vi "Set Goal D.vi"(11 "GIC Input":T1={"     Use ?\nOff       On"=[FALSE, TRUE, FALSE, TRUE], "Mode:"=FALSE, "Extra Port"="", "Hokuyo Port"="COM7", "Tx Prop  Port"="COM6", "Compass Port"="", "GPS Port"="", "Num of WPs"=0, "WP Lats and Longs"={"WP Lats"=[], "WP Longs"=[]}, "Obst Lats and Longs"={"Obst Lats"=[], "Obst Longs"=[]}, "Parameters"=[], "GPS Data"=[], "Compass"=0.0, "LMS Vector"=[], "Vision Vector"=[], "Direction Cmd"=0.0, "Speed Cmd"=0.0, "WP Vector"=[], "WP Number"=0, "Extra"=0, "SW Map"=[], "Path Cluster"={"Path x node"=[], "Path y node"=[]}, "Sim Course"=[]} {"Obst Lats and Longs"."Obst Longs" format="%#_8g"; "Obst Lats and Longs"."Obst Lats" format="%#_8g"}) -> (3 "GIC Output":T1={"     Use ?\nOff       On"=[FALSE, TRUE, FALSE, TRUE], "Mode:"=FALSE, "Extra Port"="", "Hokuyo Port"="COM7", "Tx Prop  Port"="COM6", "Compass Port"="", "GPS Port"="", "Num of WPs"=0, "WP Lats and Longs"={"WP Lats"=[], "WP Longs"=[]}, "Obst Lats and Longs"={"Obst Lats"=[], "Obst Longs"=[]}, "Parameters"=[], "GPS Data"=[], "Compass"=0.0, "LMS Vector"=[], "Vision Vector"=[], "Direction Cmd"=0.0, "Speed Cmd"=0.0, "WP Vector"=[], "WP Number"=0, "Extra"=0, "SW Map"=[], "Path Cluster"={"Path x node"=[], "Path y node"=[]}, "Sim Course"=[]} {"Obst Lats and Longs"."Obst Longs" format="%#_8g"; "Obst Lats and Longs"."Obst Lats" format="%#_8g"})   [LabVIEW 2014]
panel:
  out "tes10":dbl
  out "tes9":dbl
  out "tes8":dbl
  out "tes7":dbl
  out "tes6":dbl
  out "tes5":dbl
  out "tes4":dbl
  out "tes3":dbl
  out "tes2":dbl
  out "tes1":dbl
  out "Slant Conf":dbl
  out "Slant":dbl
  out "test 2":dbl
  out "tp":dbl
  out "wp vector":dbl[](array[numeric])
  out "test 1":dbl
  out "goal y":dbl
  out "goal x":dbl
  out "Test Output SWMap":dbl[][](array[numeric])
  # "Set Goal D"
  # "Input:"
  # "Output:"
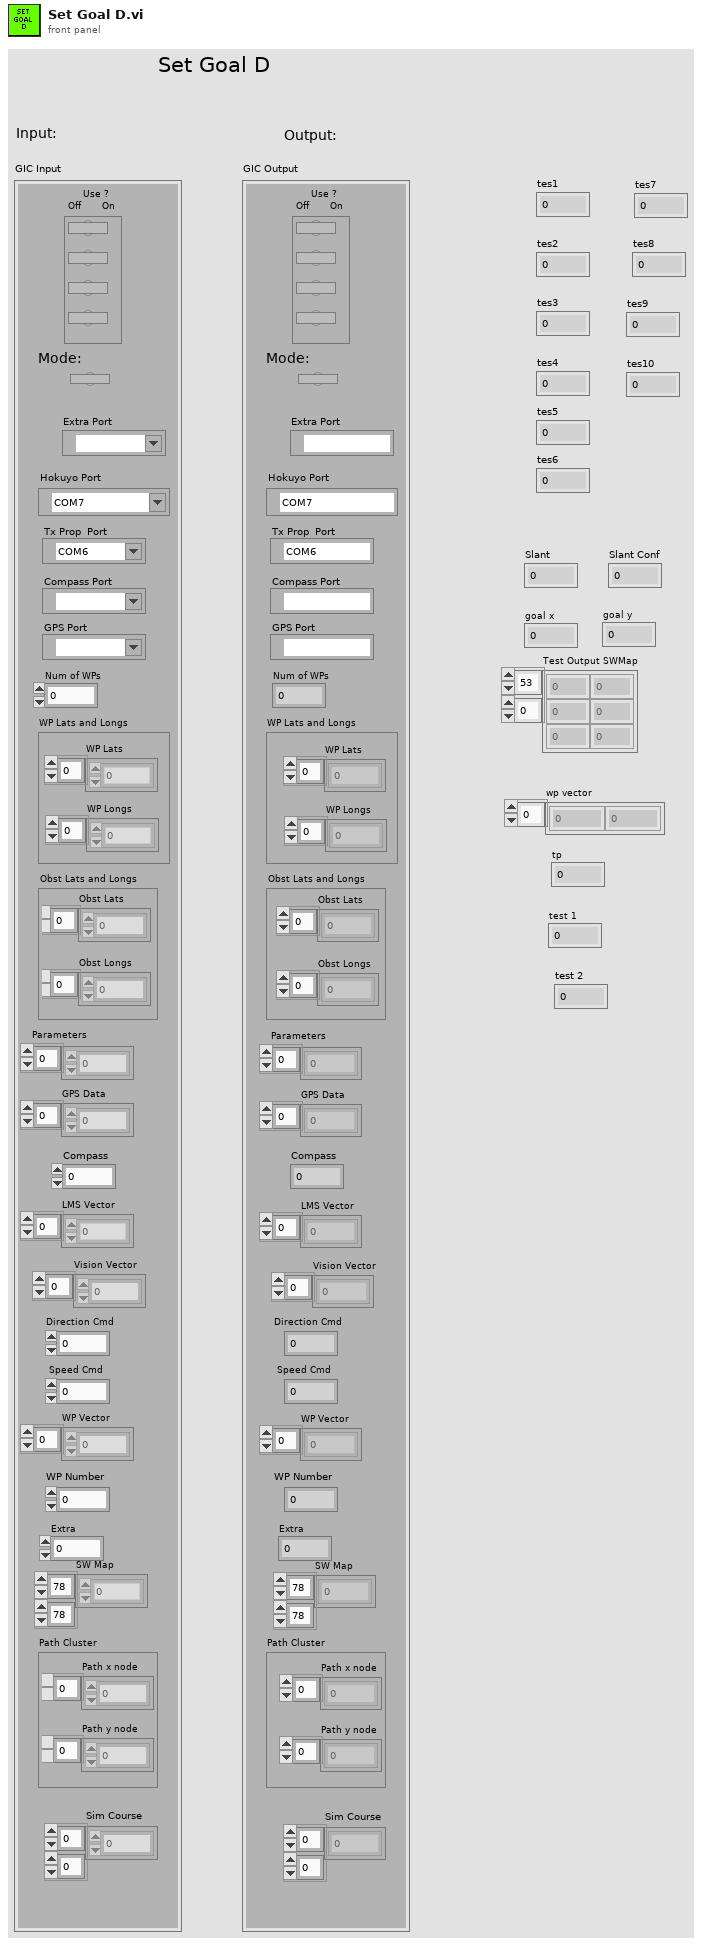
[diagram p1: front panel]
types:
  T1 = cluster{"     Use ?\nOff       On":bool[], "Mode:":bool, "Extra Port":refnum<visa-resource-name>, "Hokuyo Port":refnum<visa-resource-name>, "Tx Prop  Port":refnum<visa-resource-name>, "Compass Port":refnum<visa-resource-name>, "GPS Port":refnum<visa-resource-name>, "Num of WPs":i16, "WP Lats and Longs":cluster{"WP Lats":dbl[], "WP Longs":dbl[]}, "Obst Lats and Longs":cluster{"Obst Lats":dbl[], "Obst Longs":dbl[]}, "Parameters":dbl[], "GPS Data":dbl[], "Compass":dbl, "LMS Vector":dbl[], "Vision Vector":dbl[], "Direction Cmd":dbl, "Speed Cmd":dbl, "WP Vector":dbl[], "WP Number":i32, "Extra":i16, "SW Map":i32[][], "Path Cluster":cluster{"Path x node":dbl[], "Path y node":dbl[]}, "Sim Course":i8[][]}
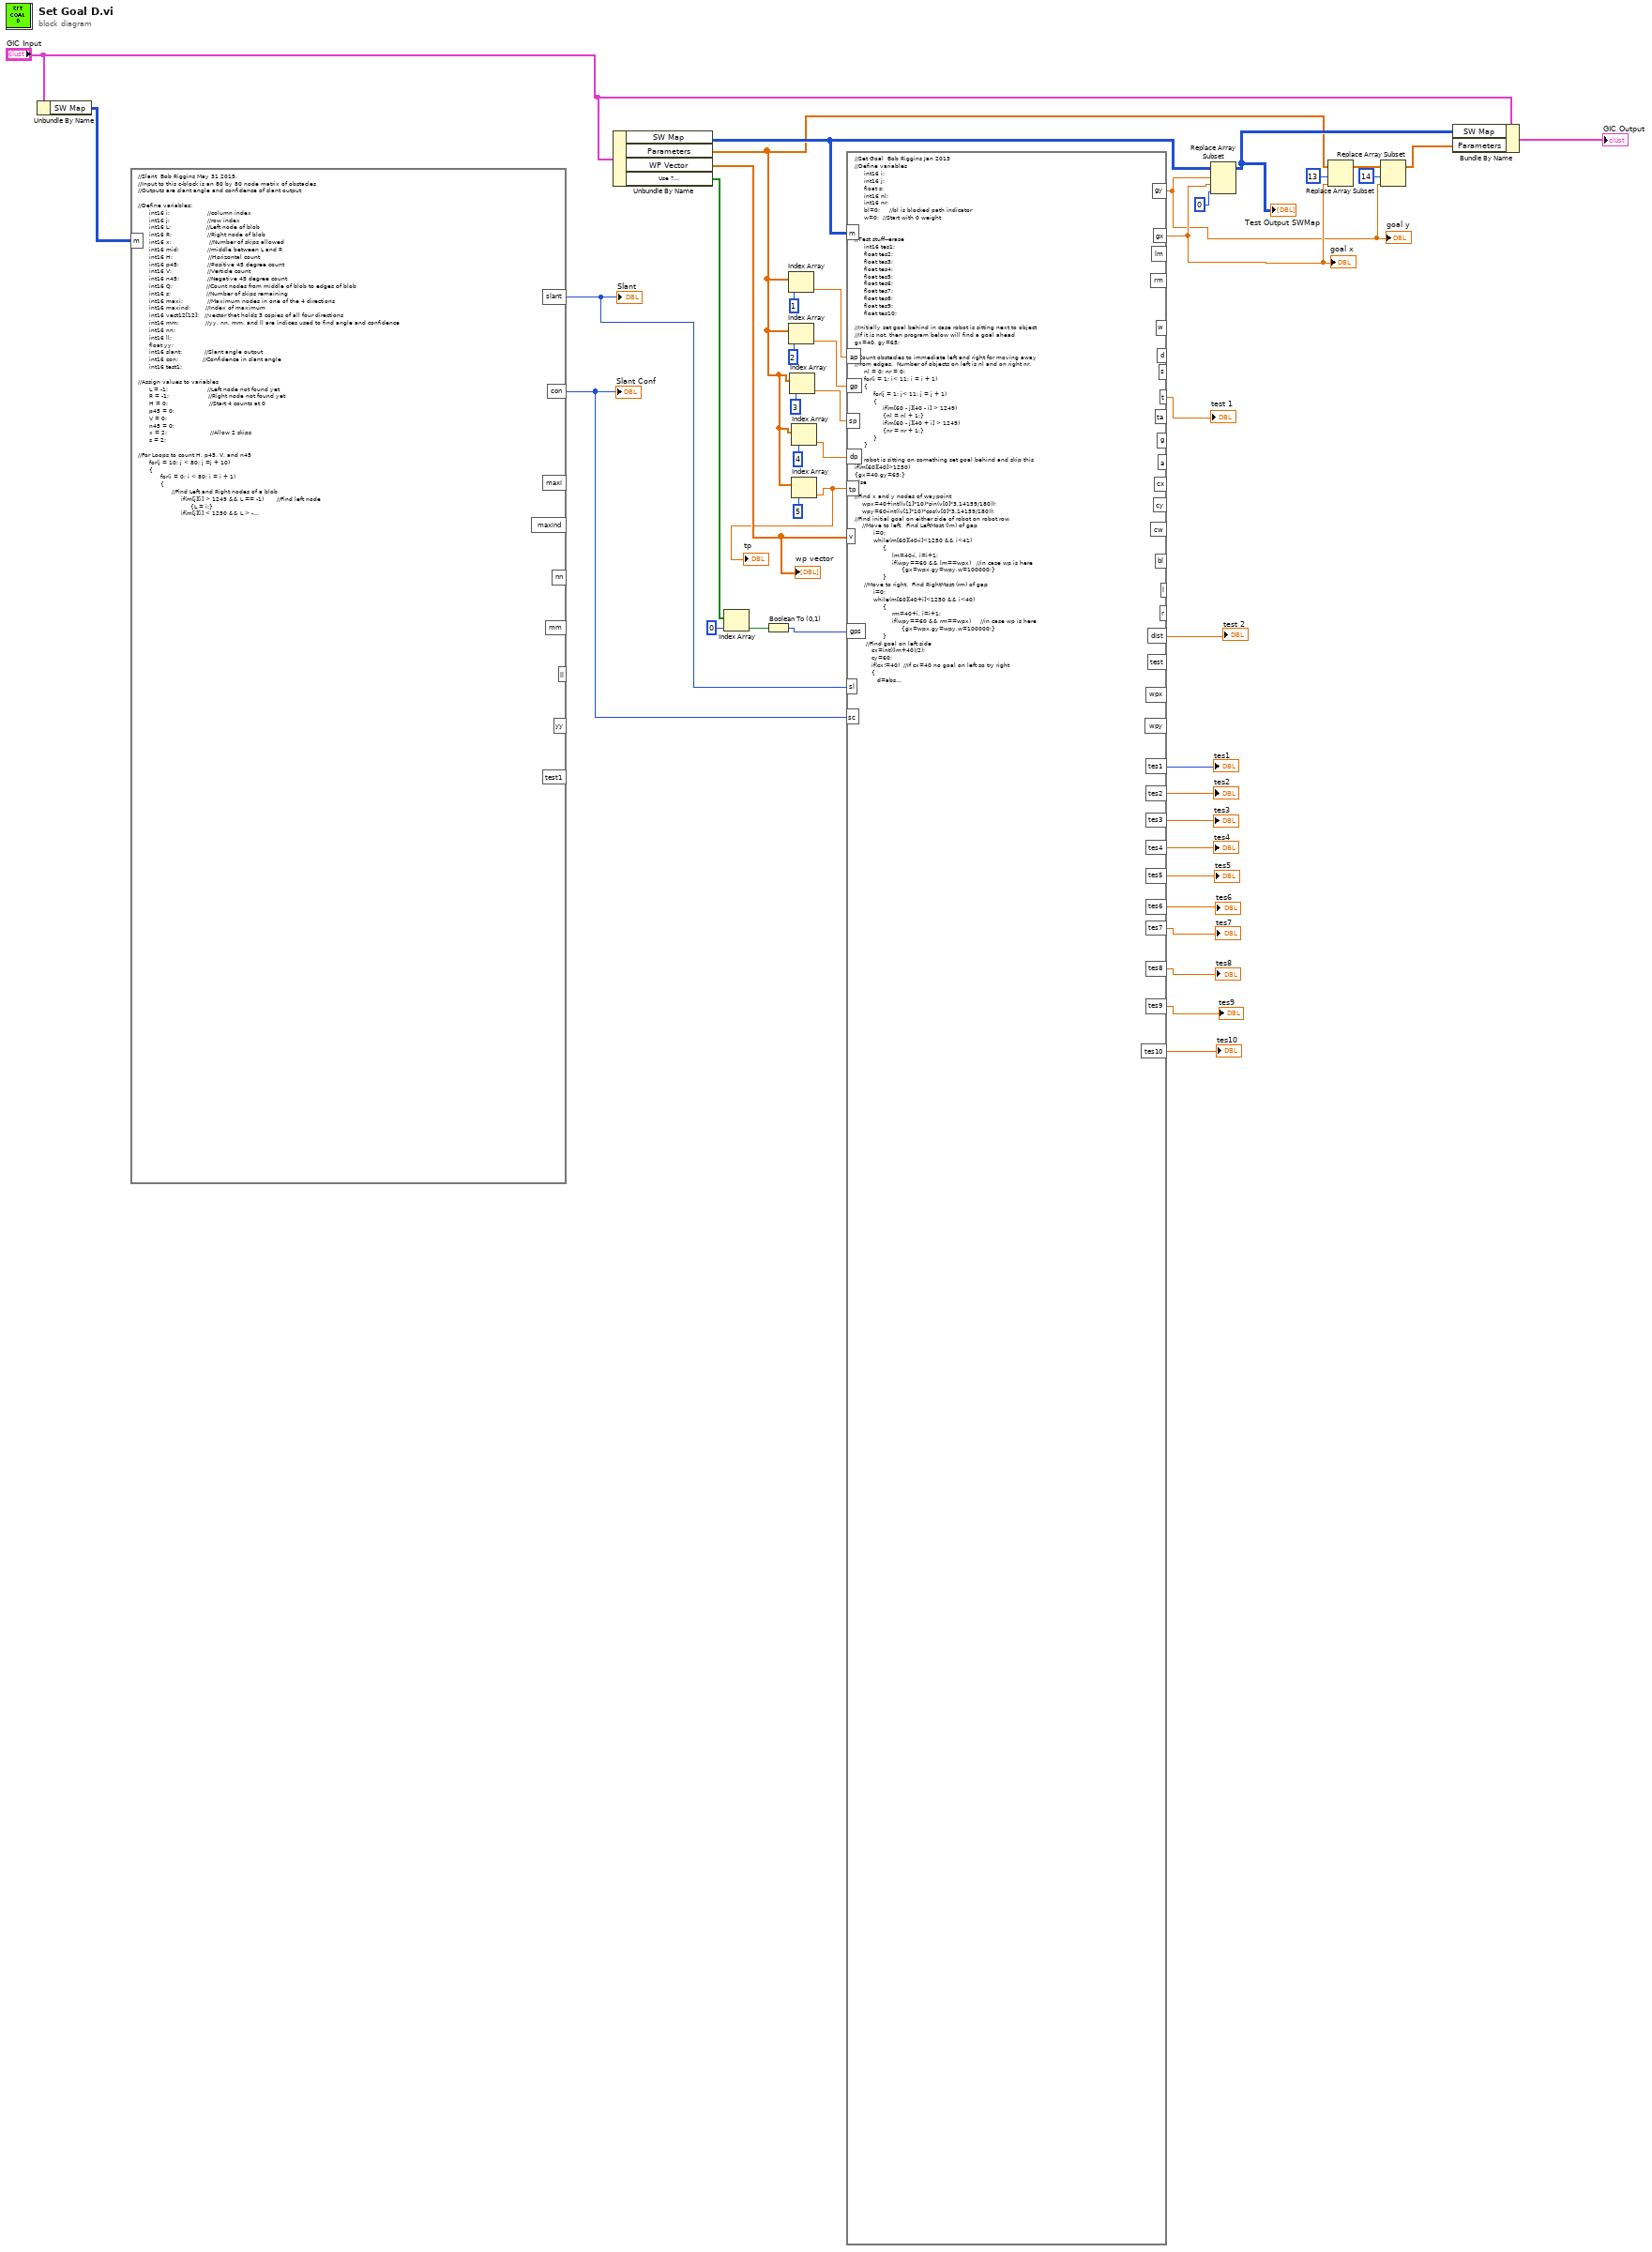
[diagram p0: block diagram]
diagram:
  n1 = Unbundle By Name("GIC Input") -> ("SW Map"=w13:i32[][])
  n2 = formula code="//Slant  Bob Riggins May 31 2015.  \n//Input to this c-block is an 80 by 80 node matrix of obstacles\n//Outputs are slant angle and confidence of slant output\n\n//Define variables:\n      int16 i;                    //column index\n      int16 j;                    //row index\n      int16 L;                   //Left node of blob\n      int16 R;                   //Right node of blob\n      int16 x;                    //Number of skips allowed\n      int16 mid;               //middle between L and R\n      int16 H;                   //Horizontal count\n      int16 p45;               //Positive 45 degree count\n      int16 V;                   //Verticle count\n      int16 n45;               //Negative 45 degree count\n      int16 Q;                  //Count nodes from middle of blob to edges of blob\n      int16 s;                   //Number of skips remaining\n      int16 maxi;             //Maximum nodes in one of the 4 directions\n      int16 maxind;        //Index of maximum\n      int16 vect12[12];   //vector that holds 3 copies of all four directions\n      int16 mm;              //yy, nn, mm, and ll are indices used to find angle and confidence\n      int16 nn;\n      int16 ll;\n      float yy;\n      int16 slant;            //Slant angle output\n      int16 con;             //Confidence in slant angle\n      int16 test1;\n\n//Assign values to variables\n      L = -1;                     //Left node not found yet\n      R = -1;                     //Right node not found yet\n      H = 0;                      //Start 4 counts at 0\n      p45 = 0;\n      V = 0;\n      n45 = 0;\n      x = 2;                       //Allow 2 skips\n      s = 2;\n\n//For Loops to count H, p45, V, and n45\n      for(j = 10; j < 80; j =j + 10)\n      {\n            for(i = 0; i < 80; i = i + 1)\n            {\n                  //Find Left and Right nodes of a blob\n                       if(m[j][i] > 1249 && L == -1)       //Find left node\n                            {L = i;}\n                       if(m[j][i] < 1250 && L > -1 && s == 0)          //Find right node\n                            {R = i - 1 - x;} \n                       if(m[j][i] <1250 && L > -1 && s > 0)         //Allow for skips\n                            {s = s - 1;}\n                       if(i == 79 && m[j][i] > 1249 && L == -1)      //single node at edge\n                       {                                                                            //define L and R there\n                             L == 79;\n                             R == 79;\n                       }       \n                       if(i == 79 && m[j][i] > 1249 && L > -1)       //blob at edge (L found)\n                            {R = 79;}   \n                       if(i == 79 && m[j][i] < 1250 && L > -1)       //blob at edge (L found)\n                            {R = 78;}\n\n                       if(L > -1 && R > -1)         //If L and R exist then start counting from mid\n                       {\n                            H = H + (R - L);                         //Updated H\n                            if(j==10)\n                                 {test1 = R;}\n                            mid = int((L + R)/2);                //Set up middle of blob for counting\n                            L = -1;\n                            R = -1;\n                            s = x;\n                            Q = 1; \n                \n                       //Count N45 (negative 45 degrees thru mid of blob)\n                            while (s > 0 && j + Q < 80 && mid + Q < 80)\n                                {\n                                     while (m[j + Q][mid + Q] > 1249)    //Count down and to right\n                                          {\n                                               n45 = n45 + 1;\n                                               s = x;\n                                               Q = Q + 1;\n                                          }\n                                     while (m[j + Q][mid + Q] < 1250 && s > 0)   //Allow x skips\n                                          {\n                                               n45 = n45 + 1;\n                                               s = s - 1;\n                                               Q = Q + 1;\n                                          }\n                                }     //end of while loop for counting n45 down and to right\n                                n45 = n45 - x;\n                                s = x;\n                                Q = 1;\n\n                                while (s > 0 && j - Q > -1 && mid - Q > -1)\n                                {\n                                     while (m[j - Q][mid - Q] > 1249)    //Count up and to left\n                                          {\n                                               n45 = n45 + 1;\n                                               s = x;\n                                               Q = Q + 1;\n                                          }\n                                     while (m[j - Q][mid - Q] < 1250 && s > 0)   //Allow x skips\n                                          {\n                                               n45 = n45 + 1;\n                                               s = s - 1;\n                                               Q = Q + 1;\n                                          }\n                                }     //end of while loop for counting n45 up and to left\n                                n45 = n45 - x;\n                                s = x;\n                                Q = 1;\n\n                       //Count V (verticle thru mid of blob)\n                            while (s > 0 && j + Q < 80)\n                                {\n                                     while (m[j + Q][mid] > 1249)    //Count down from mid\n                                          {\n                                               V = V + 1;\n                                               s = x;\n                                               Q = Q + 1;\n                                          }\n                                     while (m[j + Q][mid] < 1250 && s > 0)   //Allow x skips\n                                          {\n                                               V = V + 1;\n                                               s = s - 1;\n                                               Q = Q + 1;\n                                          }\n                                }     //end of while loop for counting V down\n                                V = V - x;\n                                s = x;\n                                Q = 1;\n\n                                while (s > 0 && j - Q > -1)\n                                {\n                                     while (m[j - Q][mid] > 1249)    //Count up\n                                          {\n                                               V = V + 1;\n                                               s = x;\n                                               Q = Q + 1;\n                                          }\n                                     while (m[j - Q][mid] < 1250 && s > 0)   //Allow x skips\n                                          {\n                                               V = V + 1;\n                                               s = s - 1;\n                                               Q = Q + 1;\n                                          }\n                                }     //end of while loop for counting V up\n                                V = V - x;\n                                s = x;\n                                Q = 1;\n\n                       //Count p45 (positive 45 degrees thru mid of blob)\n                            while (s > 0 && j + Q < 80 && mid - Q > -1)\n                                {\n                                     while (m[j + Q][mid - Q] > 1249)    //Count down and to left\n                                          {\n                                               p45 = p45 + 1;\n                                               s = x;\n                                               Q = Q + 1;\n                                          }\n                                     while (m[j + Q][mid - Q] < 1250 && s > 0)   //Allow x skips\n                                          {\n                                               p45 = p45 + 1;\n                                               s = s - 1;\n                                               Q = Q + 1;\n                                          }\n                                }     //end of while loop for counting p45 down and to left\n                                p45 = p45 - x;\n                                s = x;\n                                Q = 1;\n\n                                while (s > 0 && j - Q > -1 && mid + Q < 80)\n                                {\n                                     while (m[j - Q][mid + Q] > 1249)    //Count up and to right\n                                          {\n                                               p45 = p45 + 1;\n                                               s = x;\n                                               Q = Q + 1;\n                                          }\n                                     while (m[j - Q][mid + Q] < 1250 && s > 0)   //Allow x skips\n                                          {\n                                               p45 = p45 + 1;\n                                               s = s - 1;\n                                               Q = Q + 1;\n                                          }\n                                }     //end of while loop for counting p45 up and to right\n                                p45 = p45 - x;\n                                s = x;\n                                Q = 1;\n\n                       }                                                    //end of IF for counts for blob\n            }                                    //end of FOR for i\n      }                                          //end of FOR for j\n      \n      //Now have H, p45, V, n45.  Find slan and con  (slant angle and confidence)\n            maxi = H;                                   //Initialize process of finding maximum direction\n            maxind = 0;\n            if(p45 > maxi)\n            {\n                 maxi = p45;\n                 maxind = 1;\n            }\n            if(V > maxi)\n            {\n                 maxi = V;\n                 maxind = 2;\n            }\n            if(n45 > maxi)\n            {\n                 maxi = n45;\n                 maxind = 3;\n            }                                                    //now, max value of 4 directions in maxi\n                                                                 //maxind is index of direction of max\n\n            for(i = 0; i < 3; i = i + 1)            //Next, make vect12, 3 copies of 4 directions\n            {\n                 vect12[4*i] = H;\n                 vect12[4*i + 1] = p45;\n                 vect12[4*i + 2] = V;\n                 vect12[4*i + 3] = n45;\n            }\n           \n            if(maxi != 0)\n            {\n                 nn = vect12[maxind - 1];                          //Use max direction and \"pull\" off to sides\n                 mm = vect12[maxind + 1];\n                 ll = vect12[maxind + 2];\n                 yy = (mm - nn)/(maxi + mm + mm);\n                 con = (1 - (ll/maxi)) * 100;                                    //Confidence of slant calculation\n\n                 if(maxind == 0)                                         //Find slant angle\n                    {slant = 45 * yy;}\n                 if(maxind == 1)                                         \n                    {slant = 45 * (1 - yy);}\n                 if(maxind == 2)                                         \n                    {slant = (45 * (1 - yy)) - 45;}\n                 if(maxind == 3)                                         \n                    {slant = -45 * (1 + yy);}\n             }\n\n             if(maxi == 0)\n             {\n                  slant = 0;\n                  con = 0;\n             }"("m"=w13) -> ("slant"=w5:i16, "con"=w4:i16)  [unwired: 7 out]
  "Slant" <- w5
  "Slant Conf" <- w4
  n3 = Unbundle By Name("GIC Input") -> ("SW Map"=w40:i32[][], "Parameters"=w30:dbl[], "WP Vector"=w23:dbl[], "Use ?\nOff       On"=w21:bool[])
  "wp vector" <- w23
  n4 = Index Array(array=w21, index=0) -> (element=w19:bool)
  n5 = Boolean To (0,1)(Boolean=w19) -> (0, 1=w18:i16)
  n6 = Index Array(array=w30, index=1) -> (element=w39:dbl)
  n7 = Index Array(array=w30, index=2) -> (element=w36:dbl)
  n8 = Index Array(array=w30, index=3) -> (element=w34:dbl)
  n9 = Index Array(array=w30, index=4) -> (element=w32:dbl)
  n10 = Index Array(array=w30, index=5) -> (element=w22:dbl)
  "tp" <- w22
  n11 = formula code="//Set Goal  Bob Riggins Jan 2013\n//Define variables\n     int16 i;\n     int16 j;\n     float s;\n     int16 nl;\n     int16 nr;\n     bl=0;     //bl is blocked path indicator\n     w=0;  //Start with 0 weight\n     \n\n//Test stuff--erase\n     int16 tes1;\n     float tes2;\n     float tes3;\n     float tes4;\n     float tes5;\n     float tes6;\n     float tes7;\n     float tes8;\n     float tes9;\n     float tes10;\n\n//Initially set goal behind in case robot is sitting next to object\n//If it is not, then program below will find a goal ahead\ngx=40, gy=65;\n\n//Count obstacles to immediate left and right for moving away\n//from edges.  Number of objects on left is nl and on right nr.\n     nl = 0; nr = 0;\n     for(i = 1; i< 11; i = i + 1)\n     {\n          for(j = 1; j< 11; j = j + 1)\n          {\n               if(m[60 - j][40 - i] > 1249)\n               {nl = nl + 1;}\n               if(m[60 - j][40 + i] > 1249)  \n               {nr = nr + 1;}\n          }\n     }   \n\n//If robot is sitting on something set goal behind and skip this\nif(m[60][40]>1250)\n{gx=40,gy=65;}\nelse\n{\n//Find x and y nodes of waypoint\n    wpx=40+int((v[1]*10)*sin(v[0]*3.14159/180));\n    wpy=60-int((v[1]*10)*cos(v[0]*3.14159/180));\n//Find initial goal on either side of robot on robot row\n    //Move to left.  Find LeftMost (lm) of gap\n          i=0;\n          while(m[60][40-i]<1250 && i<41)\n               {\n                    lm=40-i, i=i+1;\n                    if(wpy==60 && lm==wpx)   //in case wp is here\n                         {gx=wpx,gy=wpy,w=100000;}\n               }\n     //Move to right.  Find RightMost (rm) of gap\n          i=0;\n          while(m[60][40+i]<1250 && i<40)\n               {\n                    rm=40+i, i=i+1;\n                    if(wpy==60 && rm==wpx)     //in case wp is here\n                         {gx=wpx,gy=wpy,w=100000;}\n               }\n      //Find goal on left side\n         cx=int((lm+40)/2);\n         cy=60;\n         if(cx!=40)  //If cx=40 no goal on left so try right\n         {\n            d=abs(cx-40)*v[1]/100; //d depends on wp dist\n            if(d>100)\n                                    {d = 100;}\n            s=0;  //slant is not allpicable initially\n            ta=v[0]*.01745;  //Angle to waypoint (target)\n            //WP angle dot product reduces for cy=60 to:\n            t=((((sin(ta)*(cx-40))/abs(cx-40))+1)*50)/v[1];  //0-100\n            //g=(40-lm)*1.25;   //gap size 0-100\n            g = 0;\n            //a=0;  //not applicable initially\n            //a=(100-(abs(cx-40)*2.5))*(100-tp)/100;\n\n            a = 0;\n            if(nl > nr && cx > 40 && cy > 30) \n                 {a = 100;}\n            if(nl < nr && cx < 40 && cy > 30) \n                 {a = 100;}\n                       \n            cw=(d*dp)+(s*sp)+(t*tp)+(g*gp)+(a*ap);\n            if(cw>w)       //this is new weight if better than old\n              {w=cw, gx=cx, gy=cy;\n                tes1 = cx; tes2 = v[1]; tes3 = ta; tes4 = t; tes5 = g; tes6 = a;\n                tes7 = d;}\n         }\n      //Note if cx=40  no good on left so keep w=0 and try right\n      //Find candidate goal on right side\n         cx=int((40+rm)/2);  \n         cy=60;\n         if(cx!=40)  //If cx=40 no goal on right so dont even try\n         {\n              d=abs(cx-40)*v[1]/100; \n              if(d>100)\n                                    {d = 100;} \n              s=0;  //slant is not allpicable initially\n              ta=v[0]*.01745;  //Angle to waypoint (target)\n              //WP angle dot product reduces for gy=60 to:\n              t=((((sin(ta)*(cx-40))/abs(cx-40))+1)*50)/v[1];  //0-100\n              //g=(rm-40)*1.25;   //gap size 0-100\n              g = 0;\n              //a=0;  //not applicable initially\n              //a=(100-(abs(cx-40)*2.5))*(100-tp)/100;\n              a = 0;\n              if(nl > nr && cx > 40 && cy > 30) \n                  {a = 100;}\n              if(nl < nr && cx < 40 && cy > 30) \n                  {a = 100;}\n              cw=(d*dp)+(s*sp)+(t*tp)+(g*gp)+(a*ap);\n              if(cw>w)       //change goal if the right is better\n                   {w=cw, gx=cx, gy=cy;\n                     tes1 = cx; tes2 = v[1]; tes3 = ta; tes4 = t; tes5 = g; tes6 = a;\n                     tes7 = d;} \n         }    \n\n//Main Loop, move up row by row checking candidates\n//Candidate goals are midpoints and both edges of all gaps\n     cy=60;\n     while(cy>0&&bl==0)\n     {\n      //start scout one row up and 1 to left unless on edge\n           if(lm==0)\n                {cx=0;}\n           else\n                {cx=lm-1;}\n           cy=cy-1; \n      //move scout to right until on clear node\n           while(m[int(cy)][int(cx)]>1249 && cx<80)\n                {cx=cx+1;}\n           if(cx==80||cx>rm+1)\n            {bl=1;  }   //means this row is blocked--can quit looking  \n      //move scout to left until on occupied node--make new lm\n           while(m[int(cy)][int(cx)]<1250 && cx>0 && bl==0)\n                {\n                    cx=cx-1;\n                    if(cy==wpy && cx==wpx)     //in case wp is here\n                         {gx=wpx,gy=wpy,w=100000;}\n                }\n           cx=cx+1;\n           lm=cx;       //new lm\n           l=lm;              //l is left of first gap on row\n      //Find all gaps on row by finding l and r of each\n      //l of first gap already found above (l=lm)\n           i=lm;  //start scout i at lm\n           while(i<80 && bl==0)   //move across row to find all gaps  \n                {\n                     while(m[int(cy)][i]<1250 && i<80)\n                          {\n                               i=i+1;\n                               if(cy==wpy && i==wpx)     //in case wp is here\n                                    {gx=wpx,gy=wpy,w=100000;}\n                          }\n                     if(i==80)\n                          {rm=79, r=rm;}\n                     else\n                          {r=i-1;}   //we now have l and r of this gap\n\n                     //Next search for best goal so far in this gap\n                     //Set goal only in middlepoint unless on edge and\n                     //unless use gps\n\n                     if(cy==0 && gps==1)\n                     {\n                          for(cx=l;cx<=r;cx=cx+1)\n                          {\n                               dist=((cx-40)**2+(cy-60)**2)**.5;\n                               d=dist*v[1]/100; \n                               if(d>100)\n                                    {d = 100;}\n                               ta=v[0]*.01745;  //Angle to waypoint (target)\n                               t=(((((cx-40)*sin(ta)+(60-cy)*cos(ta))/dist)+1)*50)/v[1];\n                               //g=(r-l)*1.25;   //gap size 0-100\n                               if(r-l<=60)\n                                    {g=100-(abs(r-l-30)*3.33);}\n                               else\n                                    {g=0;}\n                               a=0;  //not applicable initially \n                               //a=(100-(abs(cx-40)*2.5))*(100-tp)/100;\n                               //a = (60 - cy)*v[1]/dist;\n                               s=((((cx-40)*sin(sl*3.14159/180)+(60-cy)*cos(sl*3.14159/180))/dist)+1)*sc/2;\n                               cw=(d*dp)+(s*sp)+(t*tp)+(g*gp)+(a*ap);\n                               if(cw>w)       //change goal if it beats all before\n                                    {w=cw, gx=cx, gy=cy;\n                                      tes1 = dist; tes2 = d; tes3 = s; tes4 = a; tes5 = g; tes6 = w;\n                                      tes7 = v[0]; tes10 = t;}\n                              tes8 = l;\n                               tes9 = r;\n                          } \n                     }\n                     else\n                     {\n                          cx=int((l+r)/2);\n                          dist=((cx-40)**2+(cy-60)**2)**.5;\n                          d=dist*v[1]/100; \n                          if(d>100)\n                                    {d = 100;}\n                          ta=v[0]*.01745;  //Angle to waypoint (target)\n                          t=(((((cx-40)*sin(ta)+(60-cy)*cos(ta))/dist)+1)*50)/v[1];\n                          //g=(r-l)*1.25;   //gap size 0-100\n                          if(l>0 && r<79)\n                          {\n                               if(r-l<=60)\n                                    {g=100-(abs(r-l-30)*3.33);}\n                               else\n                                    {g=0;}\n                          }\n                          else\n                               {g=0;}\n                          //a=0;  //not applicable initially \n                          //a=(100-(abs(cx-40)*2.5))*(100-tp)/100;\n                          //a = (60 - cy)*v[1]/dist;\n                          a = 0;\n                          if(nl > nr && cx > 40 && cy > 30) \n                               {a = 100;}\n                          if(nl < nr && cx < 40 && cy > 30) \n                               {a = 100;}\n                          s=((((cx-40)*sin(sl*3.14159/180)+(60-cy)*cos(sl*3.14159/180))/dist)+1)*sc/2;\n                          cw=(d*dp)+(s*sp)+(t*tp)+(g*gp)+(a*ap);\n                          if(cw>w)       //change goal if it beats all before\n                               {w=cw, gx=cx, gy=cy;\n                                tes1 = dist; tes2 = d; tes3 = r; tes4 = l; tes5 = g; tes6 = w;\n                                      tes7 = dp; tes10 = gp;}\n                                 \n                     } \n                     cx=r;\n                     //Move scout to right to find L of next gap     \n                          while(m[int(cy)][i]>1249 && i<80)\n                               {i=i+1; }\n                     //Dont check any more gaps on row if i>rm+1\n                        if(i>rm+1)\n                             {i=80;}\n                        if(i<80)\n                             {l=i;}\n\n                }    //end of while checking for all gaps on a row\n                rm=r;   //right max is last right on row\n   }    //end of main loop moving to top of map\n   //Last thing to do: check for too much stuff in front\n   //If so, back out. This is a trap\n        if(nl > 10 && nr > 10)\n             {gx=40, gy = 70;}\n}  //End of big if to see if robot is sitting on something"("m"=w40, "ap"=w39, "gp"=w36, "sp"=w34, "dp"=w32, "tp"=w22, "v"=w23, "gps"=w18, "sl"=w5, "sc"=w4) -> ("gx"=w28:dbl, "gy"=w25:dbl, "t"=→"test 1":dbl, "dist"=→"test 2":dbl, "tes1"=→"tes1":i16, "tes2"=→"tes2":dbl, "tes3"=→"tes3":dbl, "tes4"=→"tes4":dbl, "tes5"=→"tes5":dbl, "tes6"=→"tes6":dbl, "tes7"=→"tes7":dbl, "tes8"=→"tes8":dbl, "tes9"=→"tes9":dbl, "tes10"=→"tes10":dbl)  [unwired: 17 out]
  "goal x" <- w28
  "goal y" <- w25
  n12 = Replace Array Subset(array=w40, new element=0 ("new element/subarray"), index (row)=w25, index (col)=w28) -> (w41:i32[][])
  "Test Output SWMap" <- w41
  n13 = Replace Array Subset(array=w30, new element=w28, index=13) -> (w27:dbl[])
  n14 = Replace Array Subset(array=w27, new element=w25, index=14) -> (w24:dbl[])
  n15 = Bundle By Name(cluster="GIC Input", "SW Map"=w41, "Parameters"=w24) -> (→"GIC Output":T1)
